vi "Z focus tracking.vi"(9 "Position":dbl, 10 "RS232 settings":cluster{"Portnumber":i32, "Baudrate":u16}={"Portnumber"=12, "Baudrate"=5} {"Portnumber" items=["COM1", "COM2", "COM3", "COM4", "COM5", "COM6", "COM7", "COM8", "COM9", "COM10", "COM11", "COM12", "COM13", "COM14", "COM15", "COM16", "COM17", "COM18", "COM19", "COM20", "COM21", "COM22", "COM23", "COM24", "COM25", "COM26", "COM27", "COM28", "COM29", "COM30"]; "Baudrate" items=["9600", "14400", "19200", "38400", "57600", "115200"]}) -> (1 "XY Graph":cluster{"Y":dbl[], "Y":dbl[]}(graph), 2 "center":dbl, 3 "give up?":bool)   [LabVIEW 2012]
uses:
  <vilib>/Analysis/NI_AALPro.lvlib
panel:
  out "Waveform Graph":dbl[](graph)
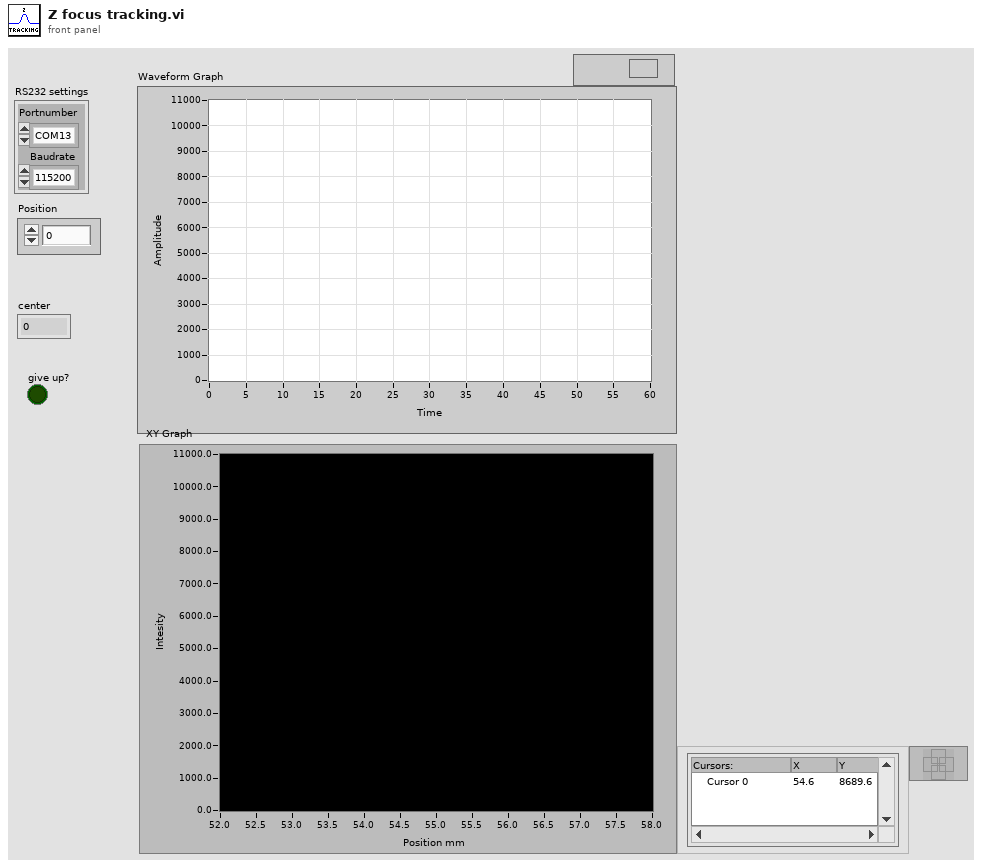
[diagram p1: front panel]
types:
  T1 = cluster{"Number of Steps":i32, "Start (mm)":dbl, "Finish (mm)":dbl}
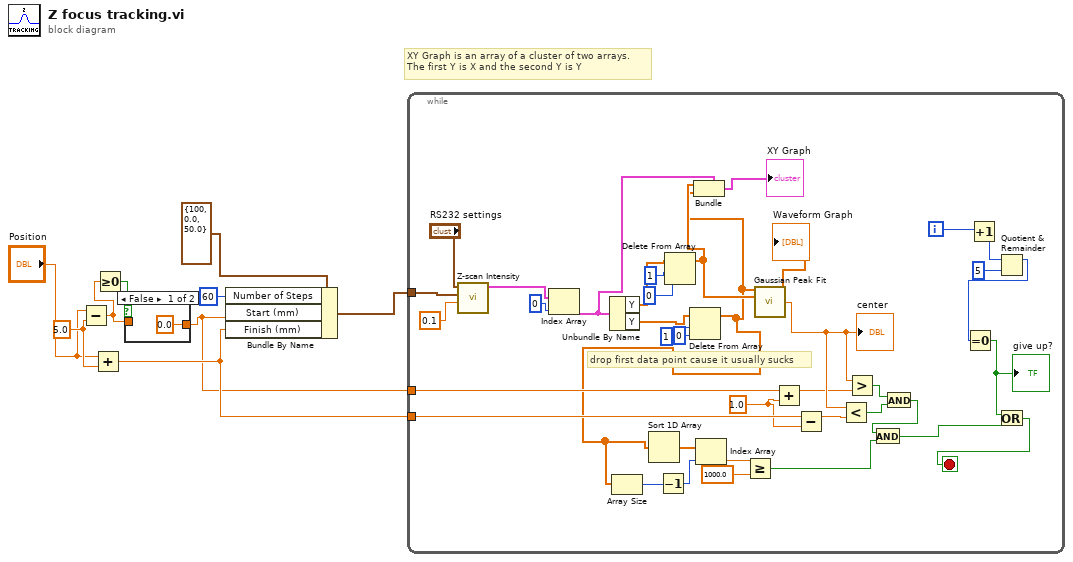
[diagram p0: block diagram]
diagram:
  w7 = 5.0 ("y")
  # "XY Graph is an array of a cluster of two arrays. \nThe first Y is X and the second Y is Y"
  n1 = Subtract(x="Position", y=w7) -> (x-y=w2:dbl)
  n2 = Add(x="Position", y=w7) -> (x+y=w4:dbl)
  n3 = Greater Or Equal To 0?(x=w2) -> (x >= 0?=w3:bool)
  n4 = case shown="False" w3 {
    tunnel: [0.0 w11] -> w1
    tunnel: w2 -> [_ w11]
    frame False {
    }
    frame True {
    }
  }
  n5 = Bundle By Name(cluster=T1 {"Number of Steps"=100, "Start (mm)"=0.0, "Finish (mm)"=50.0} ("Scan parameters"), "Number of Steps"=60, "Start (mm)"=w1, "Finish (mm)"=w4) -> (w5:T1)
  n6 = while {
    tunnel: w5 -> [w49]
    tunnel: w1 -> [w45]
    tunnel: w4 -> [w43]
    i -> [w18]
    stop <- w16 stop-if-true
    w31 = 1.0 ("y")
    # "drop first data point cause it usually sucks"
    n7 = call "Z-scan Intensity.vi"("Time Target (s)"=0.1, "Scan parameters"=w49, "RS232 settings"="RS232 settings") -> ("XY Graph"=w48:cluster{"Y":dbl[], "Y":dbl[]}[])  [unwired: 7 in, 1 out]
    n8 = Index Array(array=w48, index=0) -> (element=w24:cluster{"Y":dbl[], "Y":dbl[]})
    n9 = Unbundle By Name(w24) -> ("Y"=w28:dbl[], "Y"=w30:dbl[])
    n10 = Delete From Array(array=w28, length=1 ("index"), index=0) -> (array with subset deleted=w26:dbl[])  [unwired: 1 out]
    n11 = Delete From Array(array=w30, length=1 ("index"), index=0) -> (array with subset deleted=w25:dbl[])  [unwired: 1 out]
    n12 = Array Size(array=w25) -> (size(s)=w37:i32)
    n13 = Sort 1D Array(array=w25) -> (sorted array=w40:dbl[])
    n14 = Decrement(x=w37) -> (x-1=w36:i32)
    n15 = Bundle(cluster=w24, "Y"=w26, "Y"=w25) -> (→"XY Graph":cluster{"Y":dbl[], "Y":dbl[]})
    n16 = Index Array(array=w40, index=w36) -> (element=w39:dbl)
    n17 = Greater Or Equal?(x=w39, y=1000.0) -> (x >= y?=w34:bool)
    n18 = call <vilib>:"Gaussian Peak Fit.vi"("Y"=w25, "X"=w26) -> ("Best Gaussian Fit"=→"Waveform Graph":dbl[], "center"=w44:dbl)  [unwired: 7 in, 5 out]
    "center" <- w44
    n19 = Add(x=w45, y=w31) -> (x+y=w32:dbl)
    n20 = Subtract(x=w43, y=w31) -> (x-y=w33:dbl)
    n21 = Less?(x=w44, y=w33) -> (x < y?=w41:bool)
    n22 = Greater?(x=w44, y=w32) -> (0:w42:bool)
    n23 = And(x=w42, y=w41) -> (x .and. y?=w35:bool)
    n24 = And(x=w35, y=w34) -> (x .and. y?=w17:bool)
    n25 = Increment(x=w18) -> (x+1=w20:i32)
    n26 = Quotient & Remainder(x=w20, y=5) -> (x-y*floor(x/y)=w21:i32)  [unwired: 1 out]
    n27 = Equal To 0?(x=w21) -> (x = 0?=w19:bool)
    "give up?" <- w19
    n28 = Or(x=w19, y=w17) -> (x .or. y?=w16:bool)
  }
